vi "Do.vi"(8 "error in (no error)":errorcluster, 10 "Actor in":refnum<class "Actor.lvclass">, 11 "Configure Stop Trigger [SPT] Msg":refnum<class "Configure Stop Trigger [SPT] Msg.lvclass">) -> (0 "error out":errorcluster, 2 "Actor out":refnum<class "Actor.lvclass">)   [LabVIEW 2014, in "CS++Fgen.lvlib" / "Configure Stop Trigger [SPT] Msg.lvclass"]
doc: "This VI delivers the message to the actor by calling the appropriate method(s) on the actor."
uses:
  Configure Stop Trigger [SPT] Msg.lvclass
  <vilib>/ActorFramework/Actor/Actor.lvclass
  CS++Fgen/CS++Fgen.lvclass
  CSPP_Core/Actors/CS++PVMonitor Messages/CS++PVUpdate Msg/CS++PVUpdate Msg.lvclass/CS++PVUpdate Msg.ctl
  CSPP_Core/Classes/CS++ProcessVariables/ProcessVariable/PV.lvclass/PV.ctl
  Configure Stop Trigger [SPT] Msg.lvclass/Configure Stop Trigger [SPT] Msg.ctl
  CSPP_Core/Classes/CS++ProcessVariables/ProcessVariable/PV.lvclass
  CSPP_Core/Actors/CS++PVMonitor Messages/CS++PVUpdate Msg/CS++PVUpdate Msg.lvclass
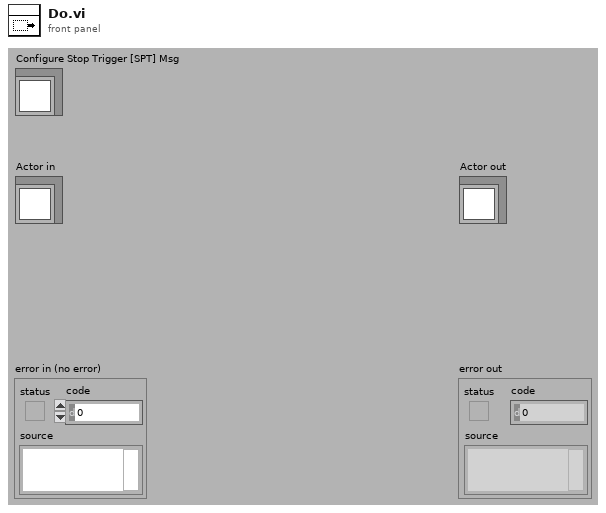
[diagram p1: front panel]
types:
  T1 = cluster{"Trigger Slope (Positive)":i32, "Channel Name (\"\")":string, "Trigger Source (None)":string}
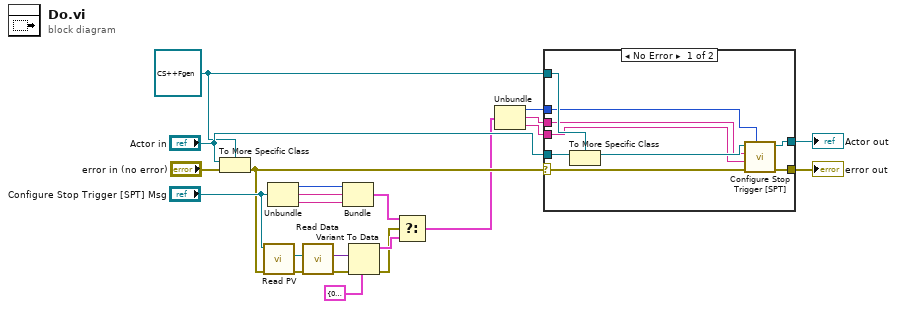
[diagram p0: block diagram]
diagram:
  w18 = refnum<class "CS++Fgen.lvclass"> refnum ("Actor in")
  n1 = To More Specific Class(target class=w18, reference="Actor in", error in="error in (no error)") -> (error out=w3:errorcluster)  [unwired: 1 out]
  n2 = call "Read PV.vi"("error in (no error)"=w3, "CS++PVUpdate Msg in"="Configure Stop Trigger [SPT] Msg") -> ("error out"=w5:errorcluster, "PV"=w14:refnum<class "PV.lvclass">)  [unwired: 7 in, 1 out]
  n3 = Unbundle("Configure Stop Trigger [SPT] Msg") -> (w8:i32, w11:string, w9:string)
  n4 = call "Read Data.vi"("error in (no error)"=w5, "PV in"=w14) -> ("error out"=w7:errorcluster, "Data"=w12:variant)  [unwired: 7 in, 1 out]
  n5 = Bundle("Trigger Slope (Positive)"=w8, "Channel Name (\"\")"=w11, "Trigger Source (None)"=w9) -> (w10:T1)  [unwired: 1 in]
  n6 = Variant To Data(error in=w7, type=T1 {"Trigger Slope (Positive)"=0, "Channel Name (\"\")"="CHANNEL1", "Trigger Source (None)"=""} ("Cluster of class private data"), Variant=w12) -> (data=w13:T1, error out=w6:errorcluster)
  n7 = Select(t=w10, s=w6, f=w13) -> (s? t:f=w2:T1)
  n8 = Unbundle(w2) -> ("Trigger Slope (Positive)"=w17:i32, "Channel Name (\"\")"=w16:string, "Trigger Source (None)"=w15:string)
  n9 = case shown="No Error" w3 {
    selector: w3 -> [w29 w33]
    tunnel: [w31 w33] -> w21
    tunnel: [w30 w32] -> w20
    tunnel: "Actor in" -> [w28 w32]
    tunnel: w18 -> [w27 _]
    tunnel: w17 -> [w25 _]
    tunnel: w16 -> [w24 _]
    tunnel: w15 -> [w23 _]
    frame No Error {
      n10 = To More Specific Class(target class=w27, reference=w28) -> (specific class reference=w26:refnum<class "CS++Fgen.lvclass">)  [unwired: 1 in, 1 out]
      n11 = call "Configure Stop Trigger [SPT].vi"("Trigger Slope (Positive)"=w25, "error in (no error)"=w29, "Trigger Source (None)"=w23, "Channel Name (\"\")"=w24, "CS++Fgen in"=w26) -> ("error out"=w31:errorcluster, "Fgen out"=w30:refnum<class "CS++Fgen.lvclass">)  [unwired: 5 in]
    }
    frame Error {
      # "If type check fails, pass the original object out again."
    }
  }
  "error out" <- w21
  "Actor out" <- w20
